vi "FlpLib ABCtoAlphaBeta_3PhaseUnitaryMagnitude 2.vi"(0 "A":sgl, 5 "B":sgl, 7 "C":sgl) -> (4 "alpha":sgl, 6 "beta":sgl)   [LabVIEW 2017]
uses:
  <userlib>/_NI FLP Library/FPGA/outsideSCTL/FlpLib Add Shared Instance 2.vi
  <userlib>/_NI FLP Library/FPGA/outsideSCTL/FlpLib Subtract Shared Instance 2.vi
  <userlib>/_NI FLP Library/FPGA/outsideSCTL/FlpLib Multiply Shared Instance 2.vi
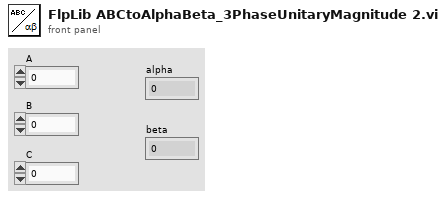
[diagram p1: front panel]
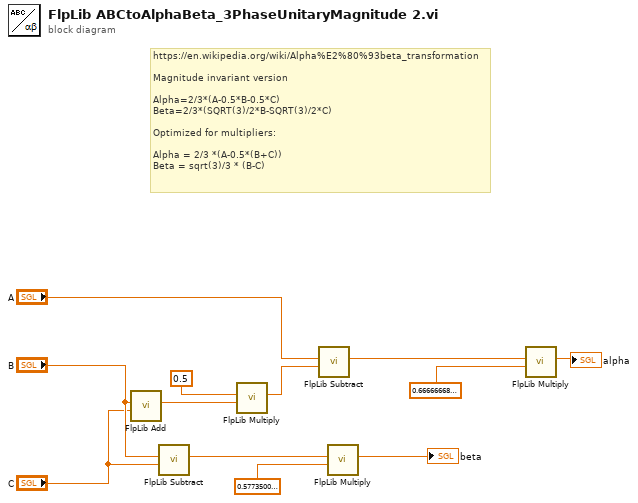
[diagram p0: block diagram]
diagram:
  # "https://en.wikipedia.org/wiki/Alpha%E2%80%93beta_transformation\n\nMagnitude invariant version\n\nAlpha=2/3*(A-0.5*B-0.5*C)\nBeta=2/3*(SQRT(3)/2*B-SQRT(3)/2*C)\n\nOptimized for multipliers:\n\nAlpha = 2/3 *(A-0.5*(B+C))\nBeta = sqrt(3)/3 * (B-C)"
  n1 = call-poly <userlib>:"FlpLib Add.vi"("y"="C", "x"="B") -> ("x+y"=w1:sgl)  [unwired: 5 in]
  n2 = call-poly <userlib>:"FlpLib Subtract.vi"("y"="C", "x"="B") -> ("x-y"=w6:sgl)  [unwired: 5 in]
  n3 = call-poly <userlib>:"FlpLib Multiply.vi"("y"=w1, "x"=sgl 0.5) -> ("x*y"=w4:sgl)  [unwired: 5 in]
  n4 = call-poly <userlib>:"FlpLib Subtract.vi"("y"=w4, "x"="A") -> ("x-y"=w8:sgl)  [unwired: 5 in]
  n5 = call-poly <userlib>:"FlpLib Multiply.vi"("y"=sgl 0.57735, "x"=w6) -> ("x*y"=→"beta":sgl)  [unwired: 5 in]
  n6 = call-poly <userlib>:"FlpLib Multiply.vi"("y"=sgl 0.6666667, "x"=w8) -> ("x*y"=→"alpha":sgl)  [unwired: 5 in]
